vi "ElmoPICtrl.vi"(8 "Actual pitch angle (rad)":dbl, 9 "Pitch setpoint (rad)":dbl, 10 "PitchCtrl":T1={"P-Gain"=0.0, "Blade pitch operating mode"=enum."Constant pitch angle", "Constant setpoint (deg)"=0.0, "Sine mean (deg)"=0.0, "Sine amp (deg)"=0.0, "Sine period (s)"=0.0, "I-Gain"=0.0, "Axis 1 On"=FALSE, "Axis 2 On"=FALSE, "Axis 3 On"=FALSE}, 11 "Axis On":bool) -> (3 "Demand out (rad/s)":dbl format="%.2f")   [LabVIEW 2018]
uses:
  Clusters/PitchCtrl.ctl
  Clusters/BladePitchMode.ctl
  <vilib>/addons/control/pid/pid.llb/PID Output Rate Limiter (DBL).vi
  <vilib>/addons/control/pid/NI_PID_pid.lvlib
  <vilib>/ptbypt/NI_PtbyPt.lvlib
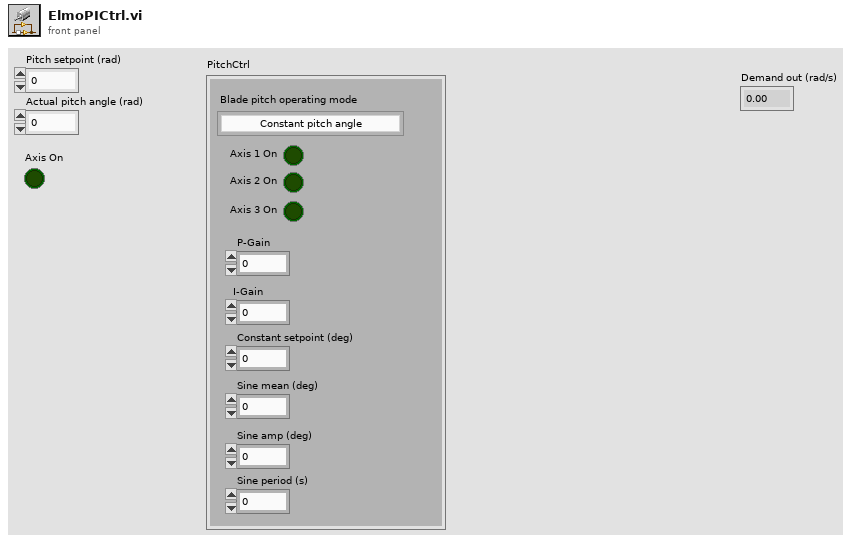
[diagram p1: front panel]
types:
  T1 = typedef "PitchCtrl.ctl" = cluster{"P-Gain":dbl, "Blade pitch operating mode":T2, "Constant setpoint (deg)":dbl, "Sine mean (deg)":dbl, "Sine amp (deg)":dbl, "Sine period (s)":dbl, "I-Gain":dbl, "Axis 1 On":bool, "Axis 2 On":bool, "Axis 3 On":bool}
  T2 = typedef "BladePitchMode.ctl" = enum16{"Zero Pitch", "Constant pitch angle", "Harmonic pitch angle", "ROSCO controlled"}
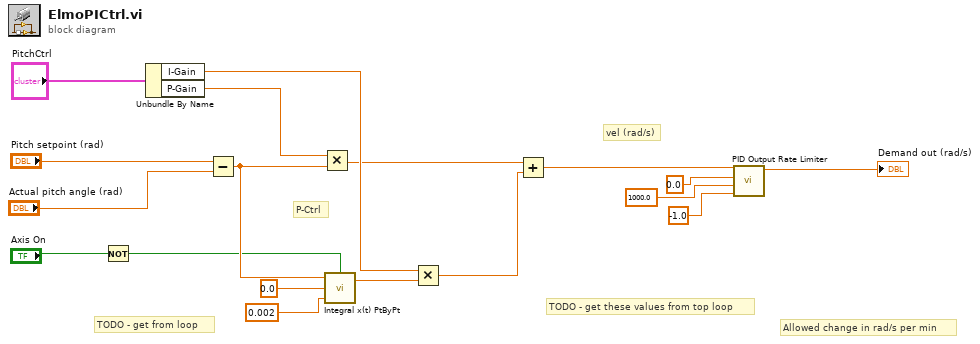
[diagram p0: block diagram]
diagram:
  # "TODO - get these values from top loop"
  # "TODO - get from loop"
  # "Allowed change in rad/s per min"
  # "P-Ctrl"
  # "vel (rad/s)"
  n1 = Not(x="Axis On") -> (.not. x?=w1:bool)
  n2 = Unbundle By Name("PitchCtrl") -> ("I-Gain"=w9:dbl, "P-Gain"=w7:dbl)
  n3 = Subtract(x="Pitch setpoint (rad)", y="Actual pitch angle (rad)") -> (x-y=w8:dbl)
  n4 = Multiply(x=w7, y=w8) -> (x*y=w6:dbl)
  n5 = call <vilib>:"Integral x(t) PtByPt.vi"("initialize"=w1, "dt"=0.002, "initial condition"=0.0, "x"=w8) -> ("integral x(t)"=w10:dbl)  [unwired: 1 out]
  n6 = Multiply(x=w9, y=w10) -> (x*y=w5:dbl)
  n7 = Add(x=w6, y=w5) -> (x+y=w4:dbl)
  n8 = call-poly <vilib>:"PID Output Rate Limiter.vi"("dt (s)"=-1.0, "output rate (EGU/min)"=1000.0, "initial output"=0.0, "input (controller output)"=w4) -> ("output"=→"Demand out (rad/s)":dbl)  [unwired: 4 in, 1 out]
